vi "CLD 13 Flow Rates Solution.vi"() -> ()   [LabVIEW 2025]
doc: "CLD 13 solution. Event driven state machine architecture. The step sequences are determined by the UI actions."
uses:
  CLD 13 State Machine Enum.ctl
  CLD 13 Data Cluster.ctl
  CLD 13 timer Enum.ctl
panel:
  out "error out":errorcluster
  in  "error in (no error)":errorcluster
  out "Flow Rate Meter":i8(knob) scale=-20.0..20.0 scale format="%_2f"
  in  "Stop Application":bool
  in  "Stop Flow":bool
  out "Elapsed Time":dbl format="%#.1g"
  out "Flow Rate":dbl
  in  "Flow Rate Change":i8(slide) min=-2 max=2 step=1 scale=-2.0..2.0
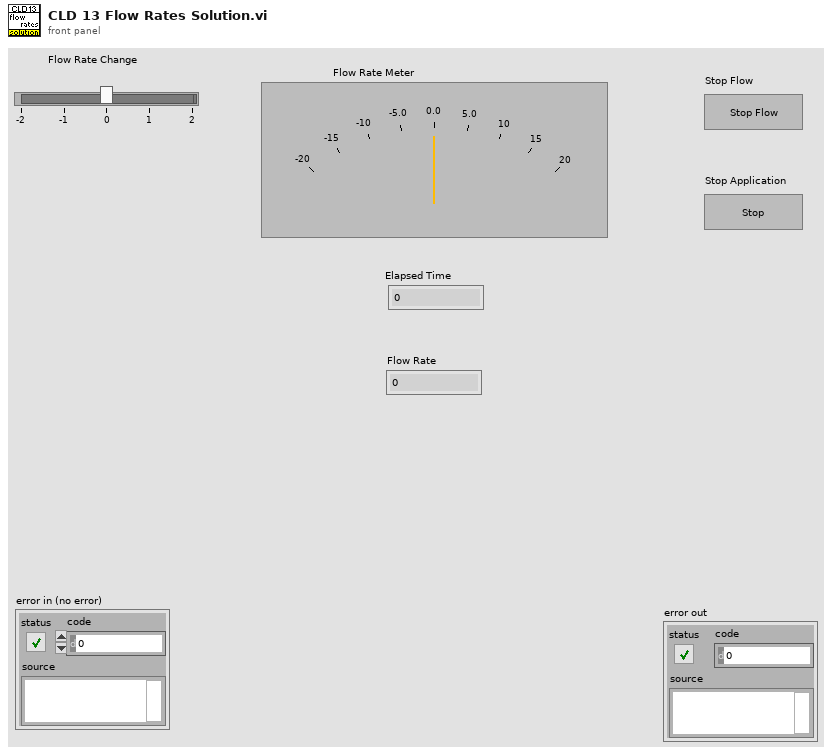
[diagram p1: front panel]
types:
  T1 = typedef "CLD 13 Data Cluster.ctl" = cluster{"Flow Rate Change":i8, "Flow Rate":i8}
  T2 = typedef "CLD 13 State Machine Enum.ctl" = enum16{"Initialize", "Idle", "Stop Flow", "Process"}
  T3 = typedef "CLD 13 timer Enum.ctl" = enum16{"Start", "Read"}
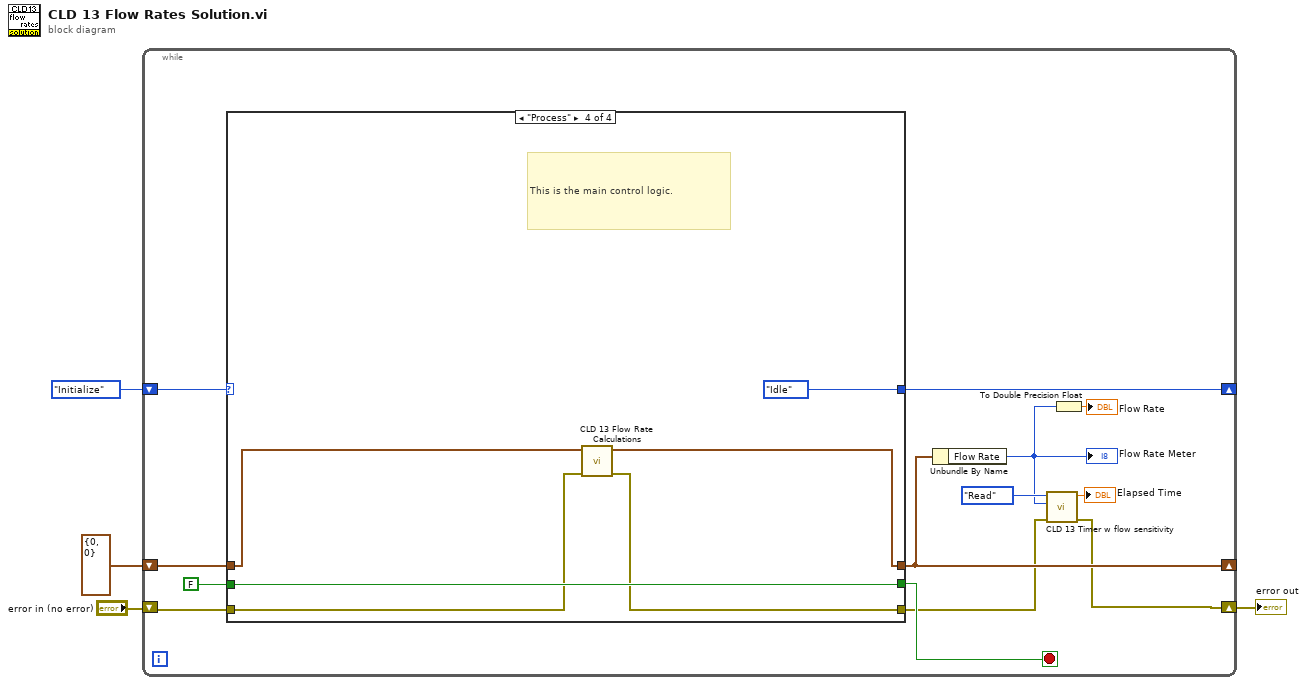
[diagram p0: block diagram]
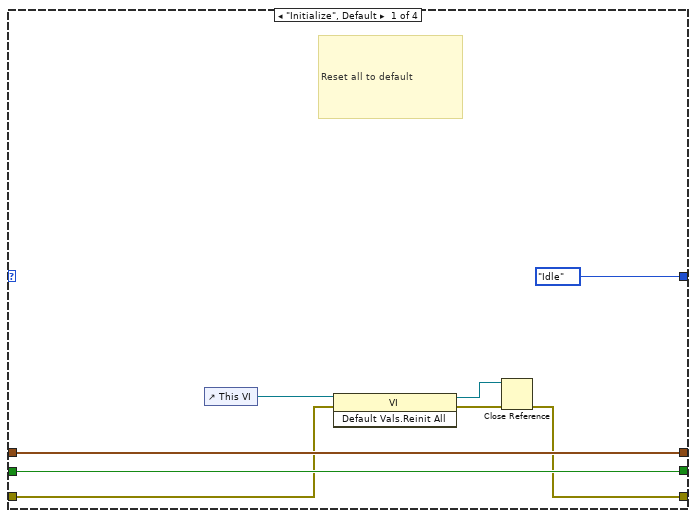
[diagram p2: hidden frame]
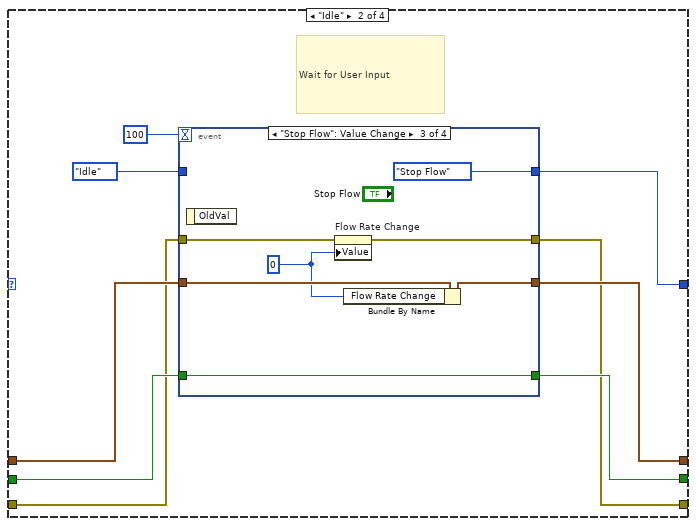
[diagram p3: hidden frame]
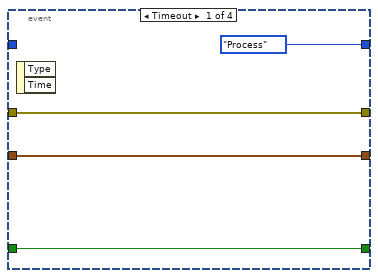
[diagram p4: hidden frame]
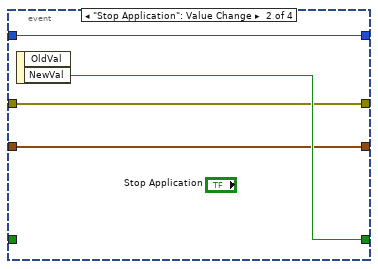
[diagram p5: hidden frame]
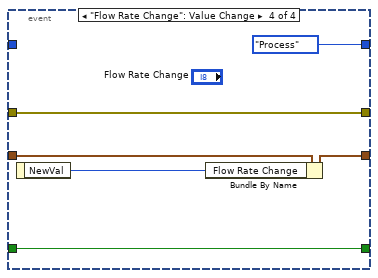
[diagram p6: hidden frame]
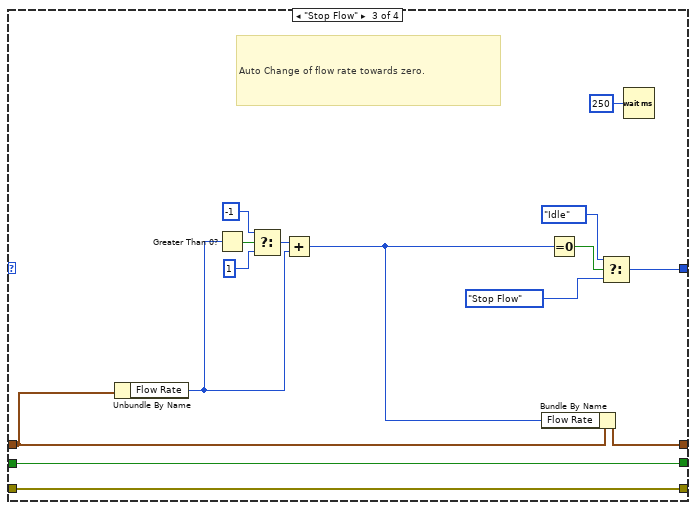
[diagram p7: hidden frame]
diagram:
  n1 = while {
    shift-right: [w14] -> _
    shift-left: CLD_13_State_Machine_Enum."Initialize" ("Enum") -> [w17]
    shift-right: [w12] -> _
    shift-left: T1 {"Flow Rate Change"=0, "Flow Rate"=0} -> [w13]
    shift-right: [w7] -> w2
    shift-left: "error in (no error)" -> [w10]
    stop <- w16 stop-if-true
    n2 = case shown="\"Process\"" w17 {
      tunnel: [w25 w33 w70 w76] -> w16
      tunnel: FALSE -> [w25 w34 w70 w76]
      tunnel: [CLD_13_State_Machine_Enum."Idle" ("Enum") w30 w60 CLD_13_State_Machine_Enum."Idle" ("Enum")] -> w14
      tunnel: w13 -> [w23 w32 w69 w75]
      tunnel: [w23 w31 w68 w74] -> w12
      tunnel: [w18 w26 w58 w71] -> w8
      tunnel: w10 -> [w19 w27 w58 w72]
      frame "Initialize", Default {
        # "Reset all to default"
        n3 = control-ref of="This VI"() -> (w20:refnum<vi>)
        n4 = invoke class="VI" method="Default Vals.Reinit All"(reference=w20, error in=w19) -> (reference out=w21:refnum<vi>, error out=w22:errorcluster)  [unwired: 1 in, 1 out]
        n5 = Close Reference(reference=w21, error in (no error)=w22) -> (error out=w18:errorcluster)
      }
      frame "Idle" {
        # "Wait for User Input"
        n6 = event shown="[2] \"Stop Flow\": Value Change" {
          selector: _ -> [_ _ _ _]
          dyn-events: _ -> [_ _ _ _]
          timeout: 100 -> [_ _ _ _]
          tunnel: w34 -> [w38 _ w48 w54]
          tunnel: [w38 w42 w48 w54] -> w33
          tunnel: w32 -> [w37 w41 w49 w51]
          tunnel: [w37 w41 w44 w55] -> w31
          tunnel: [CLD_13_State_Machine_Enum."Process" ("Enum") w40 CLD_13_State_Machine_Enum."Stop Flow" ("Enum") CLD_13_State_Machine_Enum."Process" ("Enum")] -> w30
          tunnel: CLD_13_State_Machine_Enum."Idle" ("Enum") -> [_ w40 _ _]
          tunnel: w27 -> [w35 w39 w46 w50]
          tunnel: [w35 w39 w45 w50] -> w26
          event Timeout {
            n7 = event-data() -> ()  [unwired: 1 in, 2 out]
          }
          event "Stop Application": Value Change {
            n8 = event-data() -> ("NewVal"=w42:bool)  [unwired: 1 in, 1 out]
          }
          event "Stop Flow": Value Change {
            w43 = i8 0 ("Flow Rate")
            n9 = event-data() -> ()  [unwired: 1 in, 1 out]
            n10 = property on="Flow Rate Change" class="Slide (strict)"(error in=w46, "Value"=w43) -> (error out=w45:errorcluster)  [unwired: 1 in, 1 out]
            n11 = Bundle By Name(cluster=w49, "Flow Rate Change"=w43) -> (w44:T1)
          }
          event "Flow Rate Change": Value Change {
            n12 = event-data() -> ("NewVal"=w52:i8)  [unwired: 1 in]
            n13 = Bundle By Name(cluster=w51, "Flow Rate Change"=w52) -> (w55:T1)
          }
        }
      }
      frame "Stop Flow" {
        # "Auto Change of flow rate towards zero."
        n14 = Unbundle By Name(w69) -> ("Flow Rate"=w57:i8)
        n15 = Greater Than 0?(x=w57) -> (x > 0?=w67:bool)
        n16 = Select(t=i8 -1 ("Flow Rate"), s=w67, f=i8 1 ("Flow Rate")) -> (s? t:f=w66:i8)
        n17 = Add(x=w66, y=w57) -> (x+y=w56:i8)
        n18 = Bundle By Name(cluster=w69, "Flow Rate"=w56) -> (w68:T1)
        n19 = Equal To 0?(x=w56) -> (x = 0?=w61:bool)
        n20 = Select(t=CLD_13_State_Machine_Enum."Idle" ("Enum"), s=w61, f=CLD_13_State_Machine_Enum."Stop Flow" ("Enum")) -> (s? t:f=w60:T2)
        n21 = Wait (ms)(milliseconds to wait=u32 250) -> ()  [unwired: 1 out]
      }
      frame "Process" {
        # "This is the main control logic."
        n22 = call "CLD 13 Flow Rate Calculations.vi"("Error In"=w72, "Cluster in"=w75) -> ("Error Out"=w71:errorcluster, "Cluster out"=w74:T1)  [unwired: 8 in]
      }
    }
    n23 = Unbundle By Name(w12) -> ("Flow Rate"=w5:i8)
    "Flow Rate Meter" <- w5
    n24 = call "CLD 13 Timer w flow sensitivity.vi"("Error In"=w8, "Flow Rate"=w5, "Timer Enum"=CLD_13_timer_Enum."Read") -> ("Error Out"=w7:errorcluster, "Time elapsed"=→"Elapsed Time":dbl)  [unwired: 7 in]
    n25 = To Double Precision Float(number=w5) -> (double precision float=→"Flow Rate":dbl)
  }
  "error out" <- w2
